vi "HeatingSystem_Create.vi"(0 "reference in":refnum<class "HeatingSystem.lvclass">, 2 "Rooms":T1, 5 "Error In":errorcluster) -> (14 "reference out":refnum<class "HeatingSystem.lvclass">, 19 "Error Out":errorcluster)   [LabVIEW 2024, in "HeatingSystem.lvclass"]
uses:
  HeatingSystem.lvclass
  HeatingSystem.lvclass/HeatingSystem.ctl
  House/Room_class/Room.lvclass
  Type Defs/Rooms Cluster Array.ctl
panel:
  # "Connector Pane"
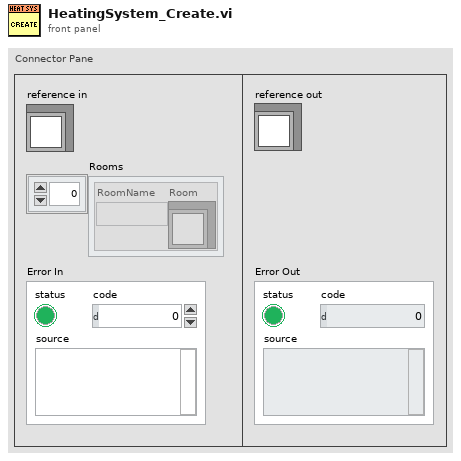
[diagram p1: front panel]
types:
  T1 = typedef "Rooms Cluster Array.ctl" = cluster{"RoomName":string, "Room":refnum<class "Room.lvclass">}[]
  T2 = typedef "HeatingSystem.lvclass/ObjectAttributes.ctl" = cluster{"Rooms":T3}
  T3 = typedef "Rooms Map.ctl" = map{string, refnum<class "Room.lvclass">}
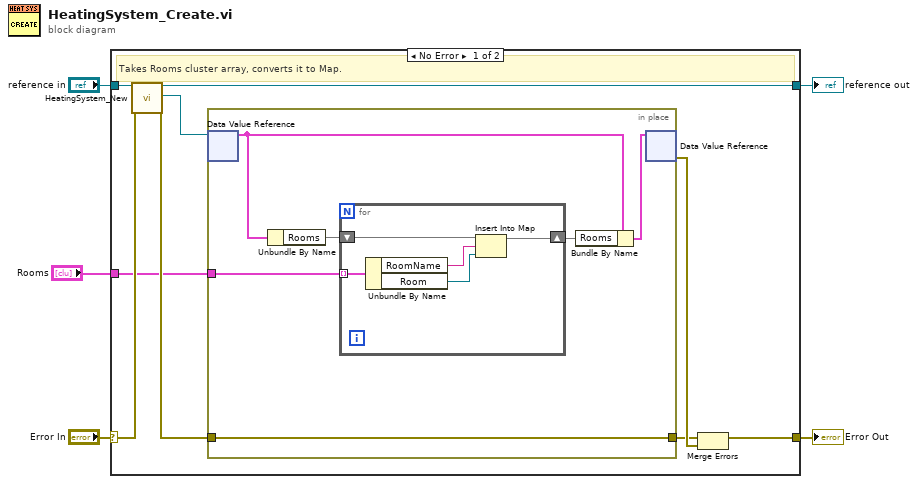
[diagram p0: block diagram]
diagram:
  n1 = case shown="No Error" "Error In" {
    selector: "Error In" -> [w13 w27]
    tunnel: [w10 w27] -> w4
    tunnel: "reference in" -> [w14 w26]
    tunnel: [w12 w26] -> w2
    tunnel: "Rooms" -> [w6 _]
    frame No Error {
      # "Takes Rooms cluster array, converts it to Map."
      n2 = call "HeatingSystem_New.vi"("reference in"=w14, "Error In"=w13) -> ("reference out"=w12:refnum<class "HeatingSystem.lvclass">, "DVRRefOut"=w9:refnum<data-value>, "Error Out"=w8:errorcluster)  [unwired: 14 in, 1 out]
      n3 = in-place {
        in-place-border: w8 -> [w20]
        in-place-border: [w20] -> w7
        in-place-border: w6 -> [w15]
        n4 = in-place-dvr #1(w9) -> (w16:T2)  [unwired: 1 out]
        n5 = Unbundle By Name(w16) -> ("Rooms"=w18:T3)
        n6 = for {
          shift-right: [w24] -> w19
          shift-left: w18 -> [w25]
          tunnel: w15 -> [w23] mode=indexing
          n7 = Unbundle By Name(w23) -> ("RoomName"=w22:string, "Room"=w21:refnum<class "Room.lvclass">)
          n8 = Insert Into Map(map in=w25, key=w22, value=w21) -> (map out=w24:T3)  [unwired: 2 out]
        }
        n9 = Bundle By Name(cluster=w16, "Rooms"=w19) -> (w17:T2)
        n10 = in-place-dvr #1(w17) -> (w11:errorcluster)  [unwired: 1 out]
      }
      n11 = Merge Errors(w7, w11) -> (w10:errorcluster)
    }
    frame Error {
      # "VI-TechBaseTemplate_Simple_6x8x6"
    }
  }
  "Error Out" <- w4
  "reference out" <- w2
